vi "Test Boolean 1D Logic.vi"() -> ()   [LabVIEW 2021]
uses:
  Source/Abs_Types/Boolean_1D/Abs_Boolean_1D.lvclass
  Source/Functions/Logic/Support/EXOR/Bool/EXOR_Bool.lvclass
  Source/Functions/Logic/Support/OR/Bool/OR_Bool.lvclass
  Source/Functions/Logic/Support/NOR/Bool/NOR_Bool.lvclass
  Source/Functions/Logic/Support/EXNOR/Bool/EXNOR_Bool.lvclass
  Source/Abs_Types/Boolean/Abs_Boolean.lvclass
  Source/Constants/Support/Bool_1D/Const_Bool_1D.lvclass
  Source/Functions/Logic/Support/AND/Bool_1D/AND_Bool_1D.lvclass
  Source/Functions/Logic/Support/NOT/Bool/NOT_Bool.lvclass
panel:
  out "EXNOR":bool
  out "NOR":bool
  out "OR":bool
  out "AND":bool[](array[boolean])
  out "EXOR":bool
  in  "Array 2":bool[](array[boolean])
  in  "Array":bool[](array[boolean])
  out "Not":bool
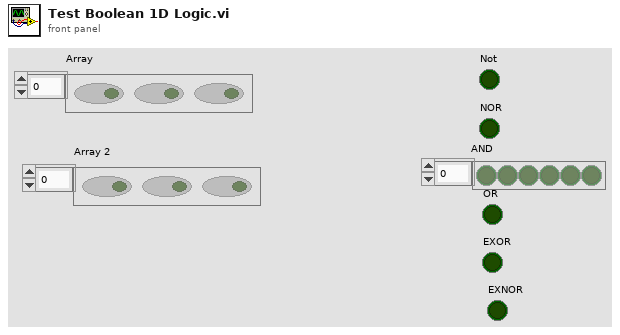
[diagram p1: front panel]
types:
  T1 = typedef "EXNOR_Bool.lvclass/Abs_Type.ctl" = refnum<class "Abs_Boolean.lvclass">
  T2 = typedef "NOR_Bool.lvclass/Abs_Type.ctl" = refnum<class "Abs_Boolean.lvclass">
  T3 = typedef "EXOR_Bool.lvclass/Abs_Type.ctl" = refnum<class "Abs_Boolean.lvclass">
  T4 = typedef "Abs_Boolean_1D.lvclass/Element Type.ctl" = bool
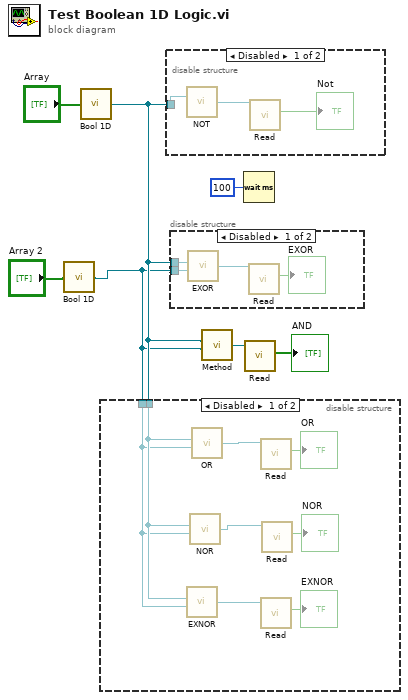
[diagram p0: block diagram]
diagram:
  n1 = call "Bool 1D.vi"("Array"="Array 2") -> ("Abs_Boolean_1D.lvclass"=w4:refnum<class "Abs_Boolean_1D.lvclass">)  [unwired: 4 in]
  n2 = call "Bool 1D.vi"("Array"="Array") -> ("Abs_Boolean_1D.lvclass"=w5:refnum<class "Abs_Boolean_1D.lvclass">)  [unwired: 4 in]
  n3 = disable-structure shown="Disabled" {
    disable-tunnel: w5 -> [w9 _]
    disable-tunnel: w4 -> [w8 _]
    frame Disabled {
      n4 = call-poly "EXNOR.vi"("B"=w8, "A"=w9) -> ("Result"=w10:T1)  [unwired: 4 in]
      n5 = call-poly "NOR.vi"("B"=w8, "A"=w9) -> ("Result"=w12:T2)  [unwired: 4 in]
      n6 = call-poly "OR.vi"("B"=w8, "A"=w9) -> ("Result"=w14:refnum<class "Abs_Boolean.lvclass">)  [unwired: 4 in]
      n7 = call-dynamic "Read.vi"("Boolean in"=w14) -> ("Boolean"=→"OR":bool)  [unwired: 8 in, 2 out]
      n8 = call-dynamic "Read.vi"("Boolean in"=w10) -> ("Boolean"=→"EXNOR":bool)  [unwired: 8 in, 2 out]
      n9 = call-dynamic "Read.vi"("Boolean in"=w12) -> ("Boolean"=→"NOR":bool)  [unwired: 8 in, 2 out]
    }
    frame Enabled {
    }
  }
  n10 = disable-structure shown="Disabled" {
    disable-tunnel: w5 -> [w18 _]
    frame Disabled {
      n11 = call-poly "NOT.vi"("Bool"=w18) -> ("Result"=w17:refnum<class "Abs_Boolean.lvclass">)  [unwired: 4 in]
      n12 = call-dynamic "Read.vi"("Boolean in"=w17) -> ("Boolean"=→"Not":bool)  [unwired: 8 in, 2 out]
    }
    frame Enabled {
    }
  }
  n13 = disable-structure shown="Disabled" {
    disable-tunnel: w5 -> [w20 _]
    disable-tunnel: w4 -> [w19 _]
    frame Disabled {
      n14 = call-poly "EXOR.vi"("B"=w19, "A"=w20) -> ("Result"=w22:T3)  [unwired: 4 in]
      n15 = call-dynamic "Read.vi"("Boolean in"=w22) -> ("Boolean"=→"EXOR":bool)  [unwired: 8 in, 2 out]
    }
    frame Enabled {
    }
  }
  n16 = call "Method.vi"("B"=w4, "A"=w5) -> ("Result"=w3:refnum<class "Abs_Boolean_1D.lvclass">)  [unwired: 4 in]
  n17 = Wait (ms)(milliseconds to wait=u32 100) -> ()  [unwired: 1 out]
  n18 = call-dynamic "Read.vi"("Boolean in"=w3) -> ("Boolean 1D"=→"AND":T4[])  [unwired: 8 in, 2 out]
